vi "Set plot names.vi"(9 "Data In (ordered by ROI index)":T1, 11 "WaveformGraph in":T6) -> (3 "WaveformGraph out":T6)   [LabVIEW 2013]
uses:
  Typedefs/Xctrl-Waveform graph ref.ctl
  Data 1.ctl
  Typedefs/Xctrl-Data array.ctl
  Typedefs/Xcrtl-Data format definition.ctl
  Typedefs/Xctl-XY data type definition.ctl
  Typedefs/Xctrl-ROI type enum.ctl
  XGrapher.xctl
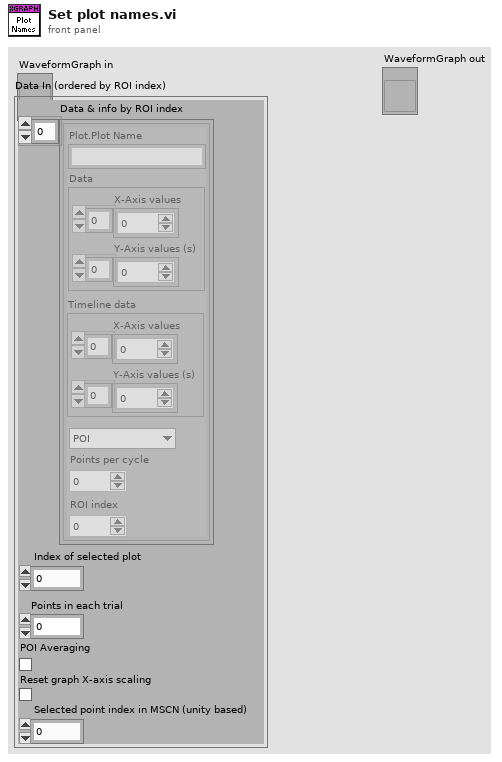
[diagram p1: front panel]
types:
  T1 = typedef "XGrapher.xctl/Data 1.ctl" = cluster{"Data & info by ROI index":T2, "Index of selected plot":u16, "Points in each trial":i32, "POI Averaging":bool, "Reset graph X-axis scaling":bool, "Selected point index in MSCN (unity based)":u16}
  T2 = typedef "Xctrl-Data array.ctl" = T3[]
  T3 = typedef "XGrapher.xctl/Xcrtl-Data format definition.ctl" = cluster{"Plot.Plot Name":string, "Data":T4, "Timeline data":T4, "Type":T5, "Points per cycle":u16, "ROI index":u16}
  T4 = typedef "XGrapher.xctl/Xctl-XY data type definition.ctl" = cluster{"X-Axis values":sgl[], "Y-Axis values (s)":i32[]}
  T5 = typedef "Xctrl-ROI type enum.ctl" = enum16{"POI", "Mini-scan", "Group"}
  T6 = typedef "XGrapher.xctl/Xctrl-Waveform graph ref.ctl" = refnum<vi>
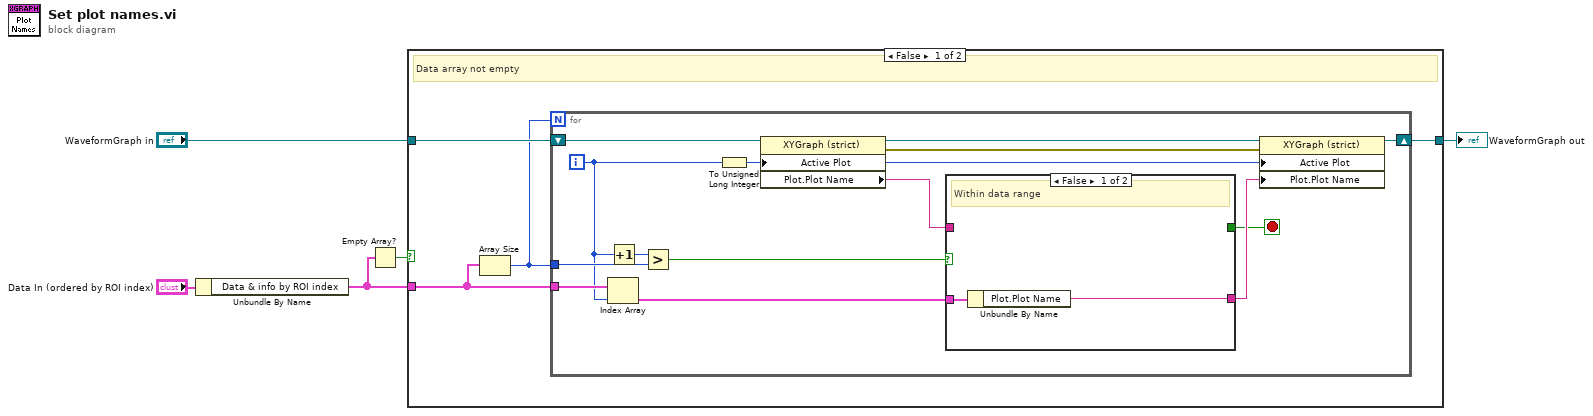
[diagram p0: block diagram]
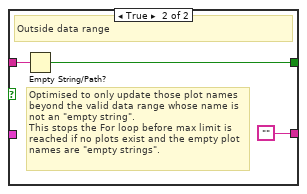
[diagram p2: hidden frame]
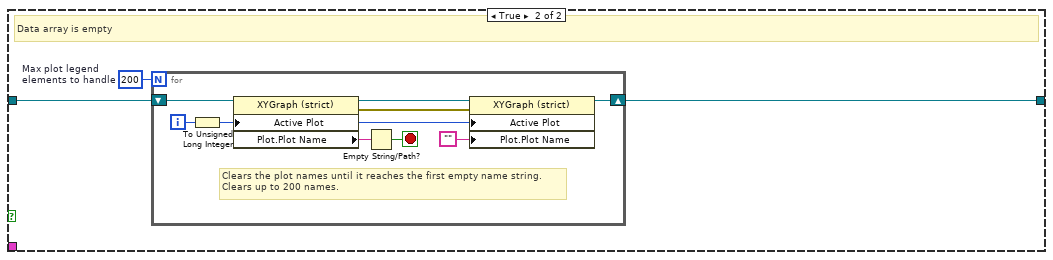
[diagram p3: hidden frame]
diagram:
  n1 = Unbundle By Name("Data In (ordered by ROI index)") -> ("Data & info by ROI index"=w1:T2)
  n2 = Empty Array?(array=w1) -> (empty?=w2:bool)
  n3 = case shown="False" w2 {
    tunnel: w1 -> [w9 _]
    tunnel: "WaveformGraph in" -> [w8 w30]
    tunnel: [w7 w29] -> w3
    frame False {
      # "Data array not empty"
      n4 = Array Size(array=w9) -> (size(s)=w6:i32)
      n5 = for {
        N: w6 -> [_]
        shift-right: [w23] -> w7
        shift-left: w8 -> [w20]
        tunnel: w9 -> [w13]
        tunnel: w6 -> [w17]
        i -> [w12]
        stop <- w15 stop-if-true
        n6 = Index Array(array=w13, index=w12) -> (element=w10:T3)
        n7 = Increment(x=w12) -> (x+1=w11:i32)
        n8 = Greater?(x=w11, y=w17) -> (0:w18:bool)
        n9 = To Unsigned Long Integer(number=w12) -> (unsigned 32bit integer=w21:u32)
        n10 = property on="Property Node" class="XYGraph (strict)"(reference=w20, "Active Plot"=w21) -> (reference out=w19:T6, error out=w14:errorcluster, "Plot.Plot Name"=w16:string)  [unwired: 1 in]
        n11 = case shown="False" w18 {
          tunnel: w10 -> [w24 _]
          tunnel: [w25 ""] -> w22
          tunnel: w16 -> [_ w27]
          tunnel: [_ w26] -> w15
          frame False {
            # "Within data range"
            n12 = Unbundle By Name(w24) -> ("Plot.Plot Name"=w25:string)
          }
          frame True {
            # "Optimised to only update those plot names beyond the valid data range whose name is not an \"empty string\".\nThis stops the For loop before max limit is reached if no plots exist and the empty plot names are \"empty strings\"."
            # "Outside data range"
            n13 = Empty String/Path?(string/path=w27) -> (empty?=w26:bool)
          }
        }
        n14 = property on="Property Node" class="XYGraph (strict)"(reference=w19, error in=w14, "Active Plot"=w21, "Plot.Plot Name"=w22) -> (reference out=w23:T6)  [unwired: 1 out]
      }
    }
    frame True {
      w31 = 200  # Max plot legend elements to handle
      # "Data array is empty"
      n15 = for {
        N: w31 -> [_]
        shift-right: [w40] -> w29
        shift-left: w30 -> [w37]
        i -> [w32]
        stop <- w34 stop-if-true
        # "Clears the plot names until it reaches the first empty name string.\nClears up to 200 names."
        n16 = To Unsigned Long Integer(number=w32) -> (unsigned 32bit integer=w38:u32)
        n17 = property on="Property Node" class="XYGraph (strict)"(reference=w37, "Active Plot"=w38) -> (reference out=w36:T6, error out=w33:errorcluster, "Plot.Plot Name"=w35:string)  [unwired: 1 in]
        n18 = Empty String/Path?(string/path=w35) -> (empty?=w34:bool)
        n19 = property on="Property Node" class="XYGraph (strict)"(reference=w36, error in=w33, "Active Plot"=w38, "Plot.Plot Name"="") -> (reference out=w40:T6)  [unwired: 1 out]
      }
    }
  }
  "WaveformGraph out" <- w3
